vi "New Frame Notify.vi"(6 "Frame Number\n(starts with 1)":i32, 8 "error in (no error)":errorcluster, 10 "Time frame start (s)":dbl, 11 "Application in":refnum<class "Application.lvclass">) -> (0 "error out":errorcluster, 3 "Application out":refnum<class "Application.lvclass">)   [LabVIEW 2018, in "Application.lvlib" / "Application.lvclass"]
uses:
  Application.lvclass
  C:/Program Files/National Instruments/LabVIEW 2018/vi.lib/ActorFramework/Actor/Actor.lvclass
  Application.lvclass/Application.ctl
  <vilib>/ActorFramework/Actor/Actor.lvclass/Actor.ctl
  <vilib>/ActorFramework/Message Enqueuer/Message Enqueuer.lvclass/Message Enqueuer.ctl
  Hardware/Stage Controller Messages/Autofocus Step Msg/Autofocus Step Msg.lvclass/Autofocus Step Msg.ctl
  <vilib>/ActorFramework/Message Enqueuer/Init from Existing Queue.vi
  <vilib>/ActorFramework/Message Enqueuer/Enqueue.vi
  Application Messages/Record Button Off Msg/Record Button Off Msg.lvclass
  C:/Program Files/National Instruments/LabVIEW 2018/vi.lib/ActorFramework/Message/Message.lvclass
  Hardware/Stage Controller Messages/Autofocus Step Msg/Autofocus Step Msg.lvclass
  Application Messages/Stop Live Mode Msg/Stop Live Mode Msg.lvclass
  Resources/GLOBAL/GLOBAL Time-critical.vi
  <vilib>/ActorFramework/Message Priority Queue/Priority Enqueue.vi
  <vilib>/ActorFramework/Message Enqueuer/Message Enqueuer.lvclass
  <vilib>/ActorFramework/Actor/Actor.lvclass
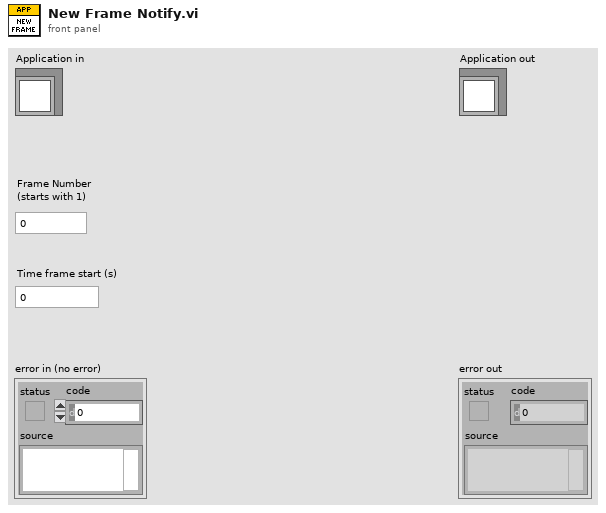
[diagram p1: front panel]
types:
  T1 = enum16{"Idle", "Live", "Stream", "Autofocus", "Z-Stack"}
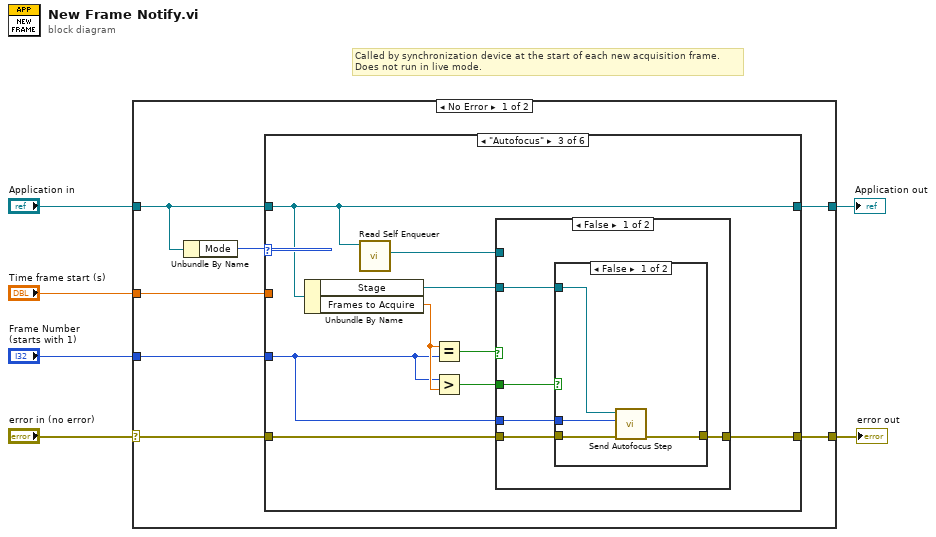
[diagram p0: block diagram]
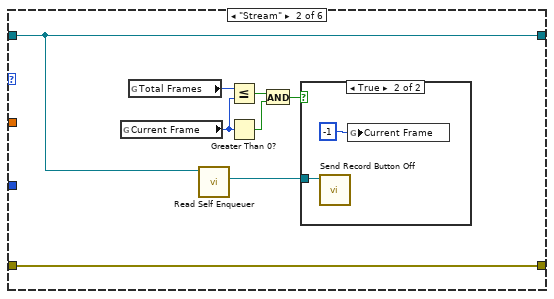
[diagram p3: hidden frame]
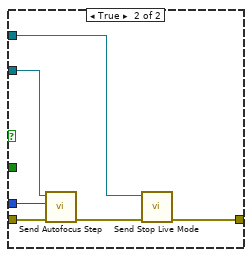
[diagram p6: hidden frame]
diagram:
  # "Called by synchronization device at the start of each new acquisition frame.\nDoes not run in live mode."
  n1 = case shown="No Error" "error in (no error)" {
    selector: "error in (no error)" -> [w9 w58]
    tunnel: [w8 w58] -> w5
    tunnel: [w7 w57] -> w3
    tunnel: "Application in" -> [w10 w57]
    tunnel: "Frame Number\n(starts with 1)" -> [w13 _]
    tunnel: "Time frame start (s)" -> [w11 _]
    frame No Error {
      n2 = Unbundle By Name(w10) -> ("Mode"=w12:T1)
      n3 = case shown="\"Autofocus\"" w12 {
        tunnel: w13 -> [_ _ w27 _ _ _]
        tunnel: w11 -> [_ _ _ _ _ _]
        tunnel: w10 -> [w14 w17 w30 w51 w53 w55]
        tunnel: w9 -> [w15 w23 w33 w52 w54 w56]
        tunnel: [w15 w23 w32 w52 w54 w56] -> w8
        tunnel: [w14 w17 w30 w51 w53 w55] -> w7
        frame Default {
        }
        frame "Stream" {
          n4 = global read "GLOBAL Time-critical.vi" "Current Frame"() -> (w18:i32)
          n5 = global read "GLOBAL Time-critical.vi" "Total Frames"() -> (w22:i32)
          n6 = call <vilib>:"Read Self Enqueuer.vi"("Actor"=w17) -> ("Self Enqueuer"=w16:refnum<class "Message Enqueuer.lvclass">)  [unwired: 10 in]
          n7 = Less Or Equal?(x=w22, y=w18) -> (x <= y?=w21:bool)
          n8 = Greater Than 0?(x=w18) -> (x > 0?=w20:bool)
          n9 = And(x=w21, y=w20) -> (x .and. y?=w19:bool)
          n10 = case shown="True" w19 {
            tunnel: w16 -> [_ w25]
            frame False {
            }
            frame True {
              n11 = call "Send Record Button Off.vi"("Message Enqueuer"=w25) -> ()  [unwired: 9 in, 2 out]
              n12 = global write "GLOBAL Time-critical.vi" "Current Frame"(-1 ("Current Frame")) -> ()
            }
          }
        }
        frame "Autofocus" {
          n13 = Unbundle By Name(w30) -> ("Stage"=w34:refnum<class "Message Enqueuer.lvclass">, "Frames to Acquire"=w28:dbl)
          n14 = call <vilib>:"Read Self Enqueuer.vi"("Actor"=w30) -> ("Self Enqueuer"=w29:refnum<class "Message Enqueuer.lvclass">)  [unwired: 10 in]
          n15 = Equal?(x=w28, y=w27) -> (x = y?=w31:bool)
          n16 = Greater?(x=w27, y=w28) -> (0:w26:bool)
          n17 = case shown="False" w31 {
            tunnel: w34 -> [w39 w49]
            tunnel: w33 -> [w38 w50]
            tunnel: [w37 w45] -> w32
            tunnel: w27 -> [w36 w48]
            tunnel: w29 -> [_ w47]
            tunnel: w26 -> [w35 _]
            frame False {
              n18 = case shown="False" w35 {
                tunnel: w39 -> [w43 _]
                tunnel: w38 -> [w42 w44]
                tunnel: [w41 w44] -> w37
                tunnel: w36 -> [w40 _]
                frame False {
                  n19 = call "Send Autofocus Step.vi"("error in (no error)"=w42, "Frame Number\n(starts with 1)"=w40, "Message Enqueuer"=w43) -> ("error out"=w41:errorcluster)  [unwired: 7 in, 1 out]
                }
                frame True {
                }
              }
            }
            frame True {
              n20 = call "Send Autofocus Step.vi"("error in (no error)"=w50, "Frame Number\n(starts with 1)"=w48, "Message Enqueuer"=w49) -> ("error out"=w46:errorcluster)  [unwired: 7 in, 1 out]
              n21 = call "Send Stop Live Mode.vi"("error in (no error)"=w46, "Message Enqueuer"=w47) -> ("error out"=w45:errorcluster)  [unwired: 8 in, 1 out]
            }
          }
        }
        frame "Z-Stack" {
        }
        frame "Live" {
        }
        frame "Idle" {
        }
      }
    }
    frame Error {
    }
  }
  "error out" <- w5
  "Application out" <- w3
